vi "ClearXYZTheta Go.vi"(8 "error in (no error)":errorcluster, 9 "Speed":dbl=100.0, 10 "XYZTheta In":dbl[](array[numeric]), 11 "Gantry In":refnum<k24>) -> (0 "error out":errorcluster, 2 "XYZTheta Out":dbl[](array[numeric]), 3 "Gantry Out":refnum<k24>)   [LabVIEW 2021, in "Motion.lvclass"]
uses:
  Motion.lvclass
  C:/Program Files (x86)/Aerotech/A3200/LabVIEW/2010/Bin/Aerotech.A3200.dll
  Program Files (x86)/Aerotech/A3200/LabVIEW/2010/Bin/Aerotech.A3200.dll
  A3200/A3200.lvclass
  Drivers/Aerotech A3200/Aerotech.lvlib
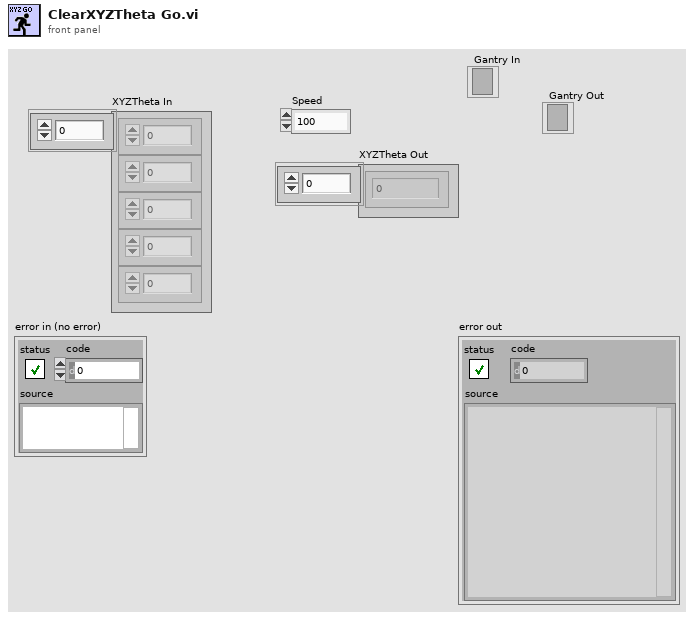
[diagram p1: front panel]
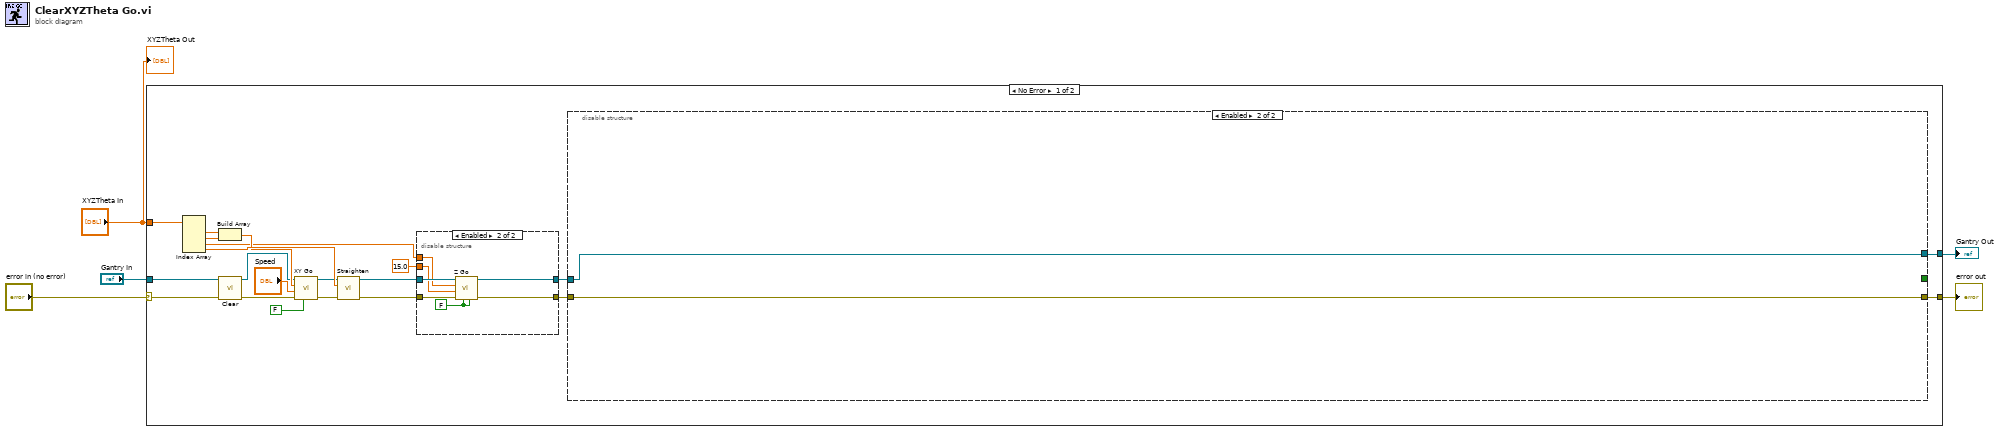
[diagram p0: block diagram]
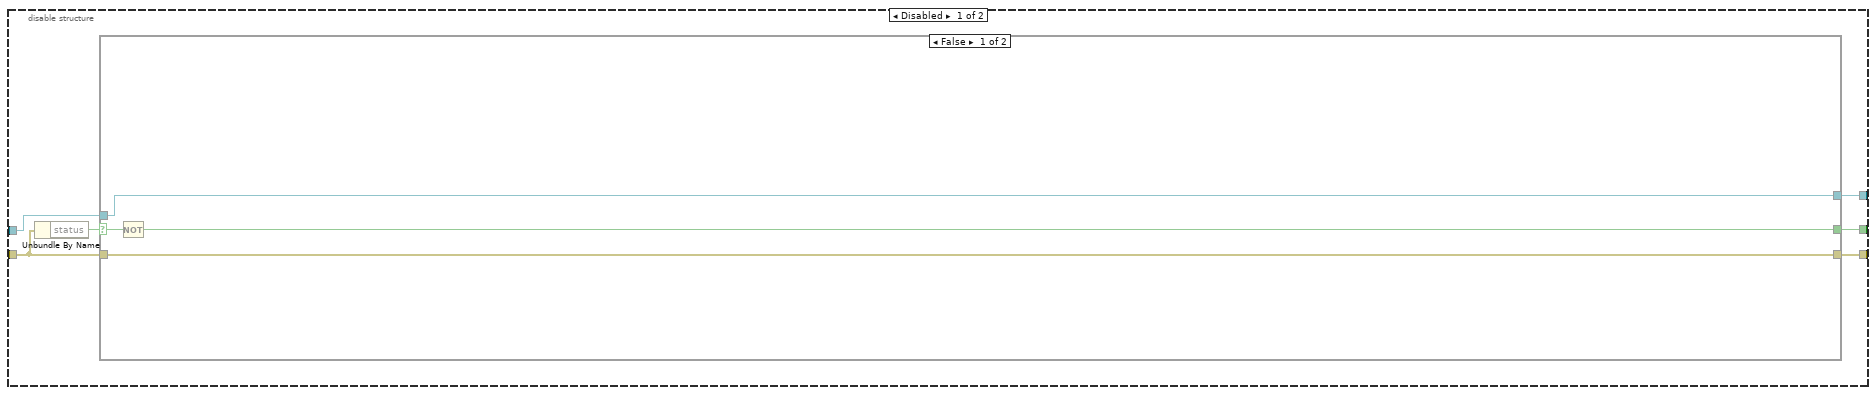
[diagram p2: hidden frame]
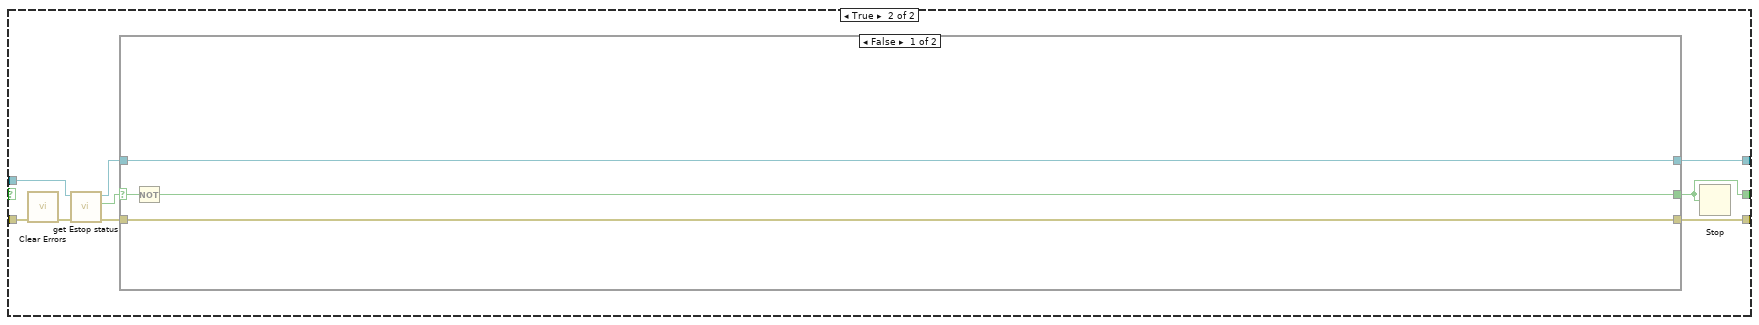
[diagram p3: hidden frame]
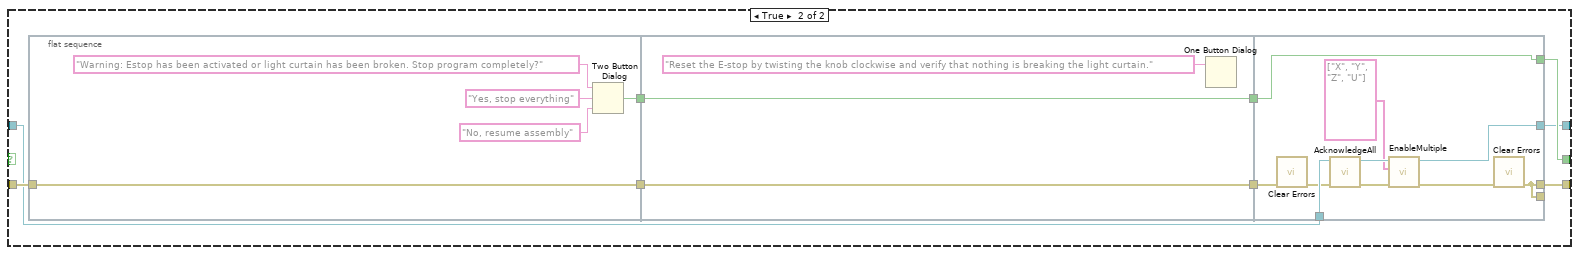
[diagram p4: hidden frame]
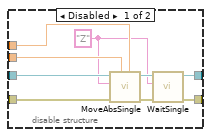
[diagram p5: hidden frame]
diagram:
  n1 = case shown="No Error" "error in (no error)" {
    selector: "error in (no error)" -> [w23 w95]
    tunnel: [w25 w95] -> w4
    tunnel: "Gantry In" -> [w24 w96]
    tunnel: [w26 w96] -> w2
    tunnel: "XYZTheta In" -> [w22 _]
    frame No Error {
      n2 = Index Array(array=w22) -> (element #1=w19:dbl, element #2=w18:dbl, element #3=w14:dbl, element #4=w21:dbl)  [unwired: 4 in]
      n3 = Build Array(w19, w18) -> (w20:dbl[])
      n4 = call "Clear.vi"("error in (no error)"=w23, "Gantry In"=w24) -> ("error out"=w11:errorcluster, "Gantry Out"=w12:refnum<k24>)  [unwired: 8 in]
      n5 = call "XY Go.vi"("return immediately"=FALSE, "error in (no error)"=w11, "Speed"="Speed", "XY In"=w20, "Gantry In"=w12) -> ("error out"=w17:errorcluster, "Gantry Out"=w9:refnum<k24>)  [unwired: 4 in, 1 out]
      n6 = call "Straighten.vi"("error in (no error)"=w17, "Angle (rad)"=w21, "Gantry In"=w9) -> ("error out"=w13:errorcluster, "Gantry Out"=w16:refnum<k24>)  [unwired: 7 in]
      n7 = disable-structure shown="Enabled" {
        disable-tunnel: w16 -> [w87 w94]
        disable-tunnel: 15.0 -> [w86 w91]
        disable-tunnel: w14 -> [w85 w92]
        disable-tunnel: w13 -> [w84 w90]
        disable-tunnel: [w82 w93] -> w6
        disable-tunnel: [w80 w88] -> w7
        frame Disabled {
          w79 = "Z" ("axis name")
          n8 = call "MoveAbsSingle.vi"("position"=w85, "speed"=w86, "error in (no error)"=w84, "axis name"=w79, "controller in"=w87) -> ("error out"=w81:errorcluster, "controller out"=w83:refnum<k24>)  [unwired: 5 in]
          n9 = call "WaitSingle.vi"("error in (no error)"=w81, "axis name"=w79, "controller in"=w83) -> ("error out"=w80:errorcluster, "controller out"=w82:refnum<k24>)  [unwired: 6 in, 1 out]
        }
        frame Enabled {
          w89 = FALSE ("Return Immediately")
          n10 = call "Z Go.vi"("Increment"=w89, "Return Immediately"=w89, "error in (no error)"=w90, "Speed In"=w91, "Position In"=w92, "Gantry In"=w94) -> ("error out"=w88:errorcluster, "Gantry Out"=w93:refnum<k24>)  [unwired: 2 in, 2 out]
        }
      }
      n11 = disable-structure shown="Enabled" {
        disable-tunnel: [w31 _] -> _
        disable-tunnel: w7 -> [w30 w77]
        disable-tunnel: [w29 w77] -> w25
        disable-tunnel: w6 -> [w28 w78]
        disable-tunnel: [w27 w78] -> w26
        frame Disabled {
          n12 = Unbundle By Name(w30) -> ("status"=w32:bool)
          n13 = case shown="False" w32 {
            selector: w32 -> [w36 _]
            tunnel: [w35 w38] -> w31
            tunnel: w30 -> [w34 w45]
            tunnel: [w34 w39] -> w29
            tunnel: w28 -> [w33 w43]
            tunnel: [w33 w37] -> w27
            frame False {
              n14 = Not(x=w36) -> (.not. x?=w35:bool)
            }
            frame True {
              n15 = call <vilib>:"Clear Errors.vi"("error in (no error)"=w45) -> ("error out"=w44:errorcluster)  [unwired: 5 in, 1 out]
              n16 = call "get Estop status.vi"("error in (no error)"=w44, "controller in"=w43) -> ("error out"=w41:errorcluster, "Estop?"=w42:bool, "controller out"=w40:refnum<k24>)  [unwired: 7 in]
              n17 = case shown="False" w42 {
                selector: w42 -> [w49 _]
                tunnel: [w48 w55] -> w38
                tunnel: w41 -> [w47 w56]
                tunnel: w40 -> [w46 w52]
                tunnel: [w47 w51] -> w39
                tunnel: [w46 w50] -> w37
                frame False {
                  n18 = Not(x=w49) -> (.not. x?=w48:bool)
                }
                frame True {
                  n19 = flat-sequence {
                    tunnel: [w63] -> w58
                    tunnel: w56 -> [w62]
                    tunnel: [w62] -> w57
                    tunnel: w58 -> [w66]
                    tunnel: w57 -> [w64]
                    tunnel: [w66] -> w54
                    tunnel: [w64] -> w53
                    tunnel: [w67] -> _
                    tunnel: [w73] -> w50
                    tunnel: [w76] -> w55
                    tunnel: w54 -> [w76]
                    tunnel: w53 -> [w75]
                    tunnel: w52 -> [w74]
                    tunnel: [w67] -> w51
                    frame #0 {
                      n20 = Two Button Dialog(message="Warning: Estop has been activated or light curtain has been broken. Stop program completely?", 1:"No, resume assembly" ("F button name (\"Cancel\")"), 2:"Yes, stop everything" ("T button name (\"OK\")")) -> (T button?=w63:bool)
                    }
                    frame #1 {
                      n21 = One Button Dialog(message="Reset the E-stop by twisting the knob clockwise and verify that nothing is breaking the light curtain.") -> ()  [unwired: 1 in, 1 out]
                    }
                    frame #2 {
                      n22 = call <vilib>:"Clear Errors.vi"("error in (no error)"=w75) -> ("error out"=w72:errorcluster)  [unwired: 5 in, 1 out]
                      n23 = call "AcknowledgeAll.vi"("error in (no error)"=w72, "controller in"=w74) -> ("error out"=w70:errorcluster, "controller out"=w71:refnum<k24>)  [unwired: 8 in]
                      n24 = call "EnableMultiple.vi"("error in (no error)"=w70, "axis names"=string[] ["X", "Y", "Z", "U"], "controller in"=w71) -> ("error out"=w68:errorcluster, "controller out"=w73:refnum<k24>)  [unwired: 7 in]
                      n25 = call <vilib>:"Clear Errors.vi"("error in (no error)"=w68) -> ("error out"=w67:errorcluster)  [unwired: 5 in, 1 out]
                    }
                  }
                }
              }
              n26 = Stop(stop? (T)=w38) -> ()
            }
          }
        }
        frame Enabled {
        }
      }
    }
    frame Error {
    }
  }
  "error out" <- w4
  "Gantry Out" <- w2
  "XYZTheta Out" <- "XYZTheta In"
